vi "xy data pin filter.vi"(0 "X-Axis Array Input":dbl[][](array[numeric])=array1024x10[10240 elements] format="%.2f", 1 "Fixed items":bool[](array[boolean]), 3 "File Info Input":T1[](array[typedef]) {"CCD Parameters"."dt or s" format="%#.6f"; "CCD Parameters"."Repetition" min=1; "CCD Parameters"."Offset" format="%#.2f"; "CCD Parameters"."Exposure Time (s)" min=0.02 max=6000.0 format="%#.2f"; "Center nm" format="%.2f"; "Temperature (K)" format="%.2f"; "Field (T)" format="%.2f"}, 5 "Data Array Input":dbl[][](array[numeric])=array1024x10[10240 elements] format="%.2f", 7 "File Info Old":T1[](array[typedef]) {"CCD Parameters"."dt or s" format="%#.6f"; "CCD Parameters"."Repetition" min=1; "CCD Parameters"."Offset" format="%#.2f"; "CCD Parameters"."Exposure Time (s)" min=0.02 max=6000.0 format="%#.2f"; "Center nm" format="%.2f"; "Temperature (K)" format="%.2f"; "Field (T)" format="%.2f"}, 9 "X-Axis Array Old":dbl[][](array[numeric])=array1024x10[10240 elements] format="%.2f", 11 "Data Array Old":dbl[][](array[numeric])=array1024x10[10240 elements] format="%.2f") -> (4 "X-Axis Array output":dbl[][](array[numeric]) format="%.2f", 8 "Data Array output":dbl[][](array[numeric]) format="%.2f", 15 "File Info Output":T1[](array[typedef]) {"CCD Parameters"."dt or s" format="%#.6f"; "CCD Parameters"."Repetition" min=1; "CCD Parameters"."Offset" format="%#.2f"; "CCD Parameters"."Exposure Time (s)" min=0.02 max=6000.0 format="%#.2f"; "Center nm" format="%.2f"; "Temperature (K)" format="%.2f"; "Field (T)" format="%.2f"})   [LabVIEW 2020]
doc: "1024x10 arrays\n10 arrays for File Info\nBoolean element in \"Fixed items\" array: true for holding \"Array old\" unchanged against \"Array Input\"; false for replacing."
uses:
  Globals and TypeDefs/Type Definitions.llb/FileInfoParameter.ctt
  Globals and TypeDefs/Type Definitions.llb/Wavelength Unit.ctt
  Globals and TypeDefs/Type Definitions.llb/McPherson Grating Density.ctl
  Globals and TypeDefs/Type Definitions.llb/CCDParameter.ctt
  Globals and TypeDefs/Type Definitions.llb/OperationMode.ctt
  Globals and TypeDefs/Type Definitions.llb/ListOfDetectors.ctt
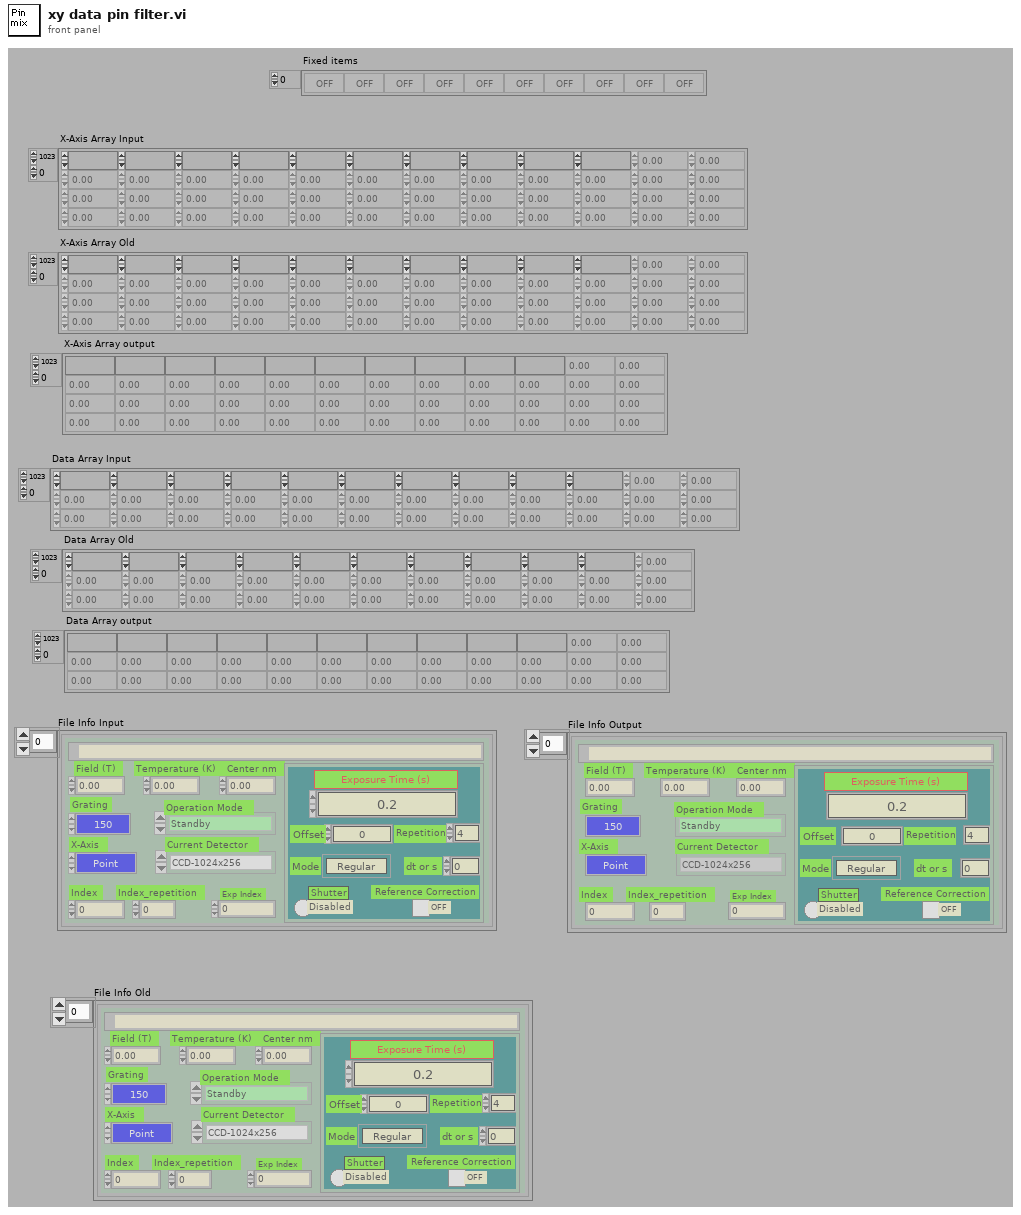
[diagram p1: front panel]
types:
  T1 = typedef "FileInfoParameter.ctt" = cluster{"FilePath":path, "Field (T)":dbl, "Temperature (K)":dbl, "X-Axis":T2, "Center nm":dbl, "Current Grating Density":T3, "CCD Parameters":T4, "Operation Mode":T5, "Exp Index":u32, "Index_repetition":u16, "Index":u16, "Current Detector":T6}
  T2 = typedef "Wavelength Unit.ctt" = enum8{"Point", "nm", "eV", "meV", "cm_1"}
  T3 = typedef "McPherson Grating Density.ctl" = enum8{"150", "300", "600", "1200", "1800"}
  T4 = typedef "CCDParameter.ctt" = cluster{"Exposure Time (s)":dbl, "Offset":dbl, "BkgrdCrct":bool, "Shutter":bool, "Mode":enum8{"Regular", "OverExp Cor", "SpikeRemove", "ForCalibration"}, "Repetition":u16, "dt or s":dbl}
  T5 = typedef "OperationMode.ctt" = enum16{"Standby", "CCD Single Shot", "CCD Sequence Shots", "CCD Custom Shots", "CCD Reference Shot", "Step Scanning ", "Time Scanning", "NML Data Acquisition"}
  T6 = typedef "ListOfDetectors.ctt" = enum8{"CCD-1024x256", "InGaAs PDA-1024x1", "CCD-1340x400", "Ge Single Channel", "Si Single Channel", "PMT Single Channel"}
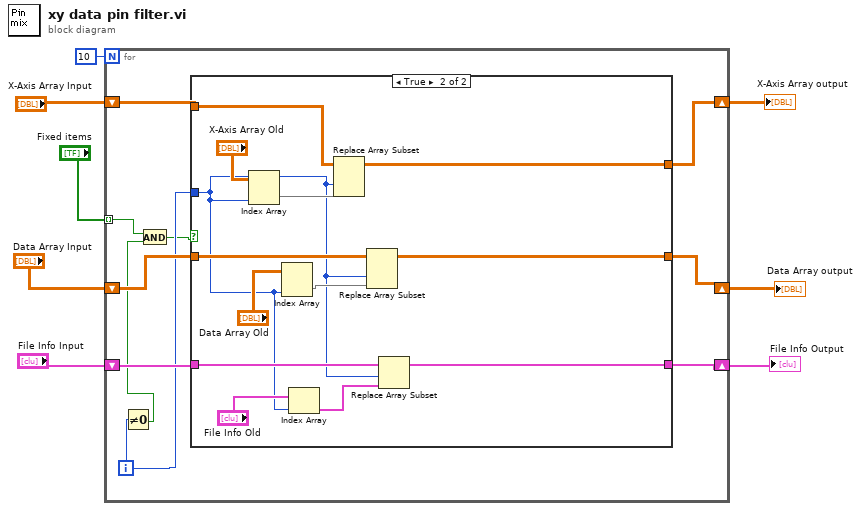
[diagram p0: block diagram]
diagram:
  n1 = for {
    N: 10 -> [_]
    tunnel: "Fixed items" -> [w10] mode=indexing
    shift-right: [w17] -> w4
    shift-left: "X-Axis Array Input" -> [w18]
    shift-right: [w16] -> w5
    shift-left: "Data Array Input" -> [w15]
    shift-right: [w13] -> w1
    shift-left: "File Info Input" -> [w14]
    i -> [w12]
    n2 = Not Equal To 0?(x=w12) -> (x != 0?=w9:bool)
    n3 = And(x=w10, y=w9) -> (x .and. y?=w11:bool)
    n4 = case shown="True" w11 {
      tunnel: w18 -> [w21 w34]
      tunnel: w12 -> [_ w22]
      tunnel: [w21 w31] -> w17
      tunnel: [w20 w30] -> w16
      tunnel: w15 -> [w20 w29]
      tunnel: w14 -> [w19 w26]
      tunnel: [w19 w25] -> w13
      frame False {
      }
      frame True {
        n5 = Index Array(array="X-Axis Array Old", index (col)=w22) -> (element=w32:dbl[])  [unwired: 1 in]
        n6 = Index Array(array="Data Array Old", index (col)=w22) -> (element=w27:dbl[])  [unwired: 1 in]
        n7 = Index Array(array="File Info Old", index=w22) -> (element=w23:T1)
        n8 = Replace Array Subset(array=w34, new element=w32, index (col)=w22) -> (w31:dbl[][])  [unwired: 1 in]
        n9 = Replace Array Subset(array=w29, new element=w27, index (col)=w22) -> (w30:dbl[][])  [unwired: 1 in]
        n10 = Replace Array Subset(array=w26, new element=w23, index=w22) -> (w25:T1[])
      }
    }
  }
  "Data Array output" <- w5
  "X-Axis Array output" <- w4
  "File Info Output" <- w1
